vi "RemplacementCaracteresInterdits.vi"(8 "error in (no error)":errorcluster, 11 "String In":string) -> (0 "error out":errorcluster, 3 "String Out":string)   [LabVIEW 2011]
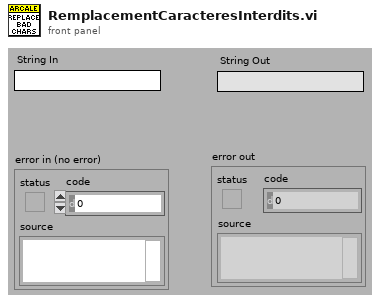
[diagram p1: front panel]
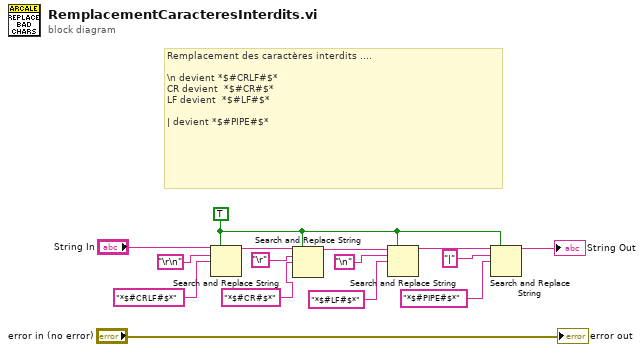
[diagram p0: block diagram]
diagram:
  w2 = TRUE ("replace all? (F)")
  # "Remplacement des caractères interdits ....\n\n\\n devient *$#CRLF#$*\nCR devient  *$#CR#$*\nLF devient  *$#LF#$*\n\n| devient *$#PIPE#$*"
  n1 = Search and Replace String(replace all?=w2, input string="String In", search string="\r\n", replace string="*$#CRLF#$*") -> (result string=w12:string)  [unwired: 4 in, 3 out]
  n2 = Search and Replace String(replace all?=w2, input string=w12, search string="\r", replace string="*$#CR#$*") -> (result string=w9:string)  [unwired: 4 in, 3 out]
  n3 = Search and Replace String(replace all?=w2, input string=w9, search string="\n", replace string="*$#LF#$*") -> (result string=w5:string)  [unwired: 4 in, 3 out]
  n4 = Search and Replace String(replace all?=w2, input string=w5, search string="|", replace string="*$#PIPE#$*") -> (result string=→"String Out":string)  [unwired: 4 in, 3 out]
  "error out" <- "error in (no error)"
